vi "Get System States.vi"(8 "error in (no error)":errorcluster, 9 "Names only?":bool, 11 "Motions in":refnum<class "Motions.lvclass">) -> (0 "error out":errorcluster, 1 "Array of Trigger State Names":string[](array[string])=["True", "False", "Move Complete", "Motion Incomplete"], 2 "States LUT (name -> boolean state)":variant, 3 "Motions out":refnum<class "Motions.lvclass">)   [LabVIEW 2016, in "Hardware.lvlib" / "Motions.lvlib" / "Motions.lvclass"]
uses:
  <userlib>/Common Components/Hardware/Abstract System/Motions/Motions/Motions.lvclass
  <userlib>/Common Components/Hardware/Abstract System/Motions/Motions/Motions.lvclass/Motions.ctl
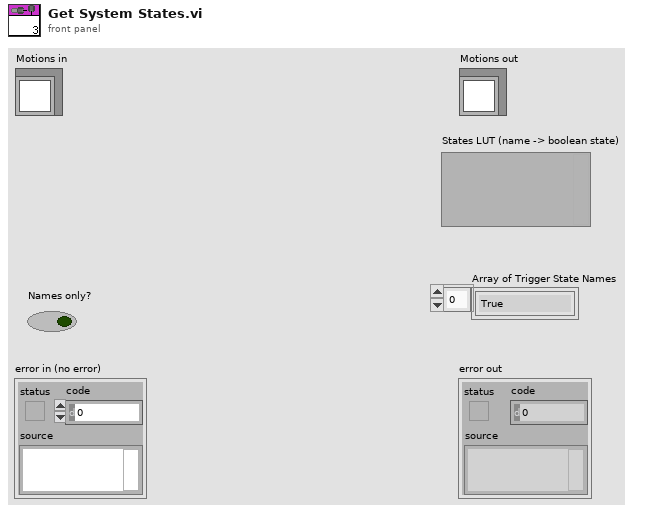
[diagram p1: front panel]
types:
  T1 = typedef "Hardware.lvlib/Motions.lvlib/Motions.lvclass/Motor States.ctl" = cluster{"Connected":bool, "Enabled":bool, "Moving Status":bool, "Soft Moving Status":bool, "Current Pos":dbl, "Target Pos":dbl, "Moving Dir (-1, 0, 1)":i32, "Error Status":bool, "Hard Limit+":bool, "Hard Limit-":bool, "Soft Limit+":bool, "Soft Limit-":bool, "History Dst Stack":refnum<queue>, "Motion Status":bool, "Motion TriggerAction Obj":refnum<class "TriggerAction Q.lvclass">}
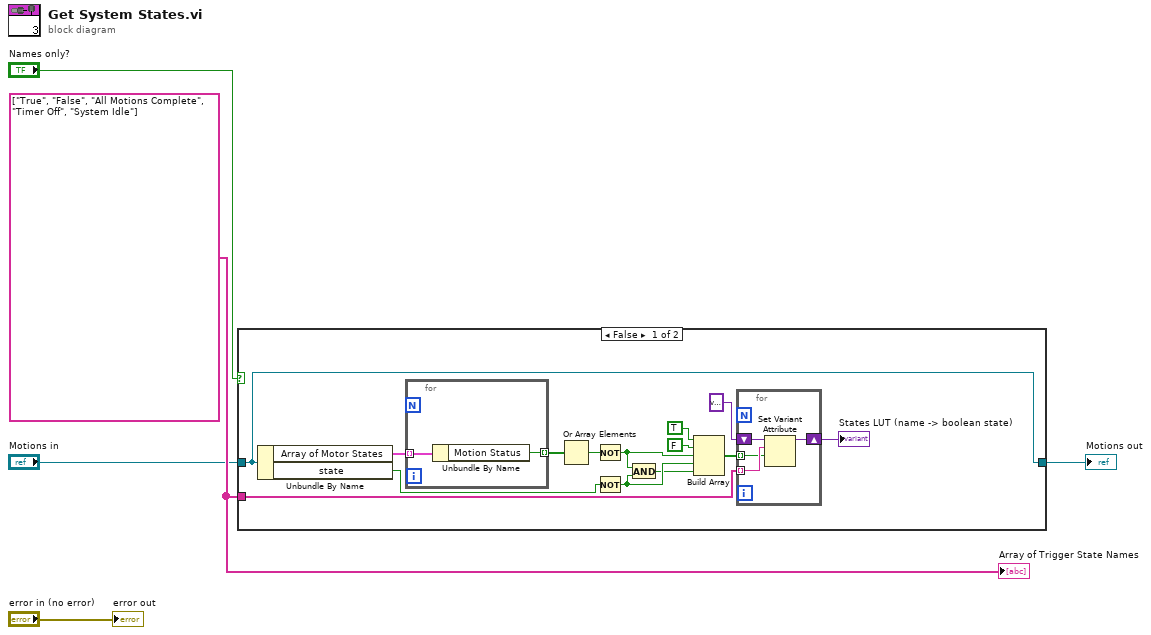
[diagram p0: block diagram]
diagram:
  w3 = string[] ["True", "False", "All Motions Complete", "Timer Off", "System Idle"] ("Array of Trigger State Names")
  n1 = case shown="False" "Names only?" {
    tunnel: w3 -> [w14 _]
    tunnel: "Motions in" -> [w6 w26]
    tunnel: [w6 w26] -> w1
    frame False {
      n2 = Unbundle By Name(w6) -> ("Array of Motor States"=w12:T1[], "state"=w13:bool)
      n3 = for {
        tunnel: w12 -> [w21] mode=indexing
        tunnel: [w20] -> w11 mode=indexing
        n4 = Unbundle By Name(w21) -> ("Motion Status"=w20:bool)
      }
      n5 = Or Array Elements(Boolean array=w11) -> (logical OR=w10:bool)
      n6 = Not(x=w10) -> (.not. x?=w9:bool)
      n7 = Not(x=w13) -> (.not. x?=w8:bool)
      n8 = And(x=w9, y=w8) -> (x .and. y?=w7:bool)
      n9 = Build Array(TRUE, FALSE, w9, w8, w7) -> (w18:bool[])
      n10 = for {
        shift-right: [w24] -> w15
        shift-left: variant -> [w25]
        tunnel: w14 -> [w23] mode=indexing
        tunnel: w18 -> [w22] mode=indexing
        n11 = Set Variant Attribute(Variant=w25, name=w23, value=w22) -> (Variant out=w24:variant)  [unwired: 1 in, 2 out]
      }
      "States LUT (name -> boolean state)" <- w15
    }
    frame True {
    }
  }
  "Motions out" <- w1
  "error out" <- "error in (no error)"
  "Array of Trigger State Names" <- w3
